vi "testAssertConnectorPanesMatchExpectedMissingFails.vi"(8 "error in (no error)":errorcluster, 11 "TestCase in":refnum<class "VeriStandTestUtilitiesTests.lvclass">) -> (0 "error out":errorcluster, 3 "TestCase out":refnum<class "VeriStandTestUtilitiesTests.lvclass">)   [LabVIEW 2027, in "VeriStandTestUtilitiesTests.lvclass"]
uses:
  VeriStandTestUtilitiesTests.lvclass
  <userlib>/_OpenG.lib/file/file.llb/Build Path - File Names Array - path__ogtk.vi
  <vilib>/addons/_JKI Toolkits/VI Tester/TestCase.llb/TestCase.lvclass
  Source/VeriStandTestUtilities/VeriStandTestUtilities.lvlib
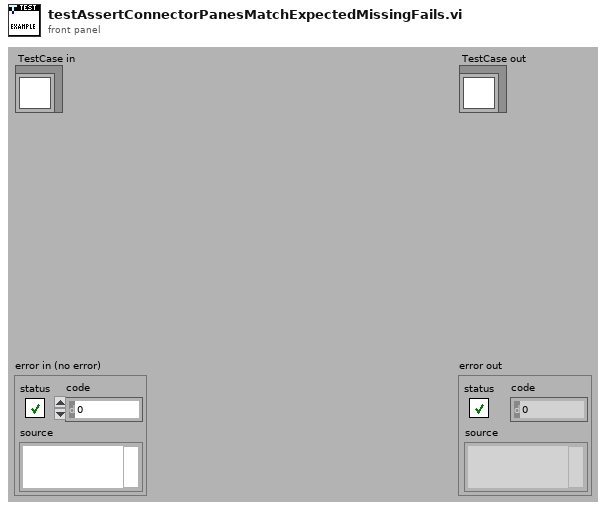
[diagram p1: front panel]
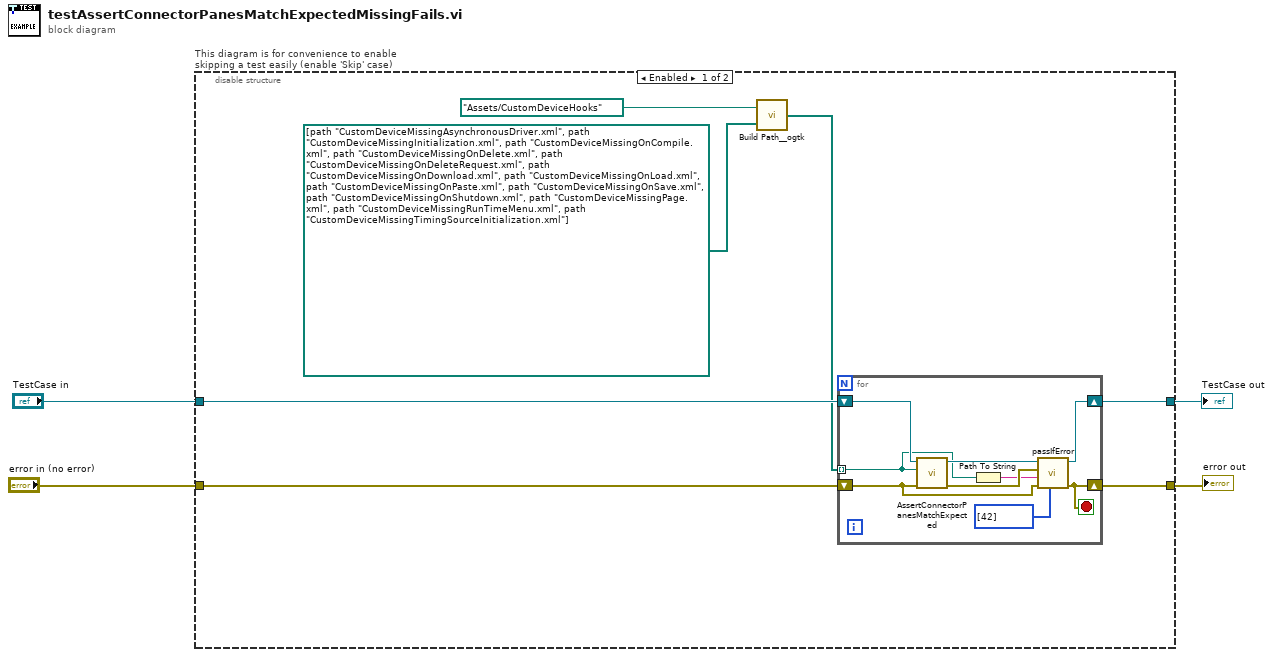
[diagram p0: block diagram]
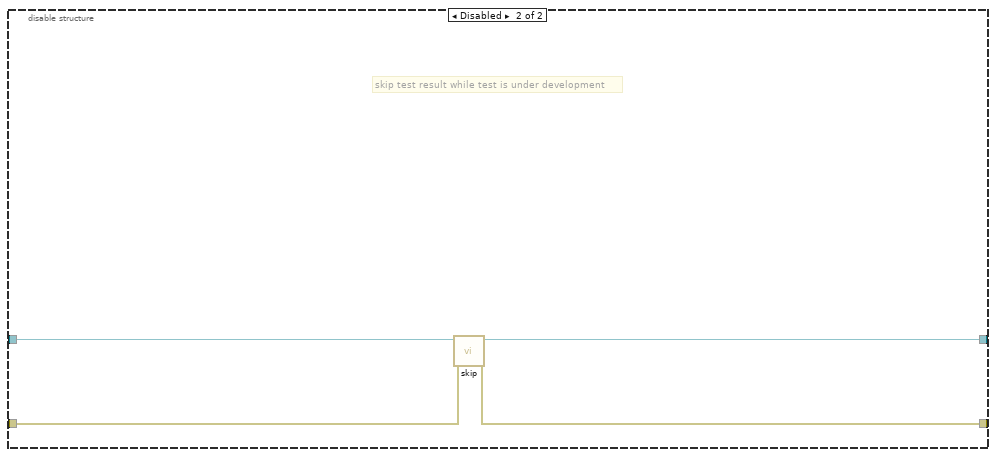
[diagram p2: hidden frame]
diagram:
  n1 = disable-structure "This diagram is for convenience to enable skipping a test easily (enable 'Skip' case)" shown="Enabled" {
    disable-tunnel: "TestCase in" -> [w9 w24]
    disable-tunnel: [w8 w22] -> w1
    disable-tunnel: [w10 w23] -> w3
    disable-tunnel: "error in (no error)" -> [w11 w21]
    frame Enabled {
      n2 = call-poly <userlib>:"Build Path__ogtk.vi"("name or relative path"=path[] [path "CustomDeviceMissingAsynchronousDriver.xml", path "CustomDeviceMissingInitialization.xml", path "CustomDeviceMissingOnCompile.xml", path "CustomDeviceMissingOnDelete.xml", path "CustomDeviceMissingOnDeleteRequest.xml", path "CustomDeviceMissingOnDownload.xml", path "CustomDeviceMissingOnLoad.xml", path "CustomDeviceMissingOnPaste.xml", path "CustomDeviceMissingOnSave.xml", path "CustomDeviceMissingOnShutdown.xml", path "CustomDeviceMissingPage.xml", path "CustomDeviceMissingRunTimeMenu.xml", path "CustomDeviceMissingTimingSourceInitialization.xml"], "base path"=path "Assets/CustomDeviceHooks") -> ("appended path"=w6:path[])
      n3 = for {
        tunnel: w6 -> [w15] mode=indexing
        shift-right: [w12] -> w10
        shift-left: w11 -> [w18]
        shift-right: [w16] -> w8
        shift-left: w9 -> [w17]
        stop <- w12 stop-if-true
        n4 = call "AssertConnectorPanesMatchExpected.vi"("error in (no error)"=w18, "custom device xml path"=w15, "TestCase in"=w17) -> ("error out"=w19:errorcluster, "TestCase out"=w20:refnum<class "VeriStandTestUtilitiesTests.lvclass">)  [unwired: 7 in]
        n5 = Path To String(path=w15) -> (string=w14:string)
        n6 = call-dynamic "passIfError.vi"("passing error codes (default = any error code)"=i32[] [42], "error in (no error)"=w18, "task (\"\")"=w14, "error"=w19, "TestCase in"=w20) -> ("error out"=w12:errorcluster, "TestCase out"=w16:refnum<class "VeriStandTestUtilitiesTests.lvclass">)  [unwired: 5 in]
      }
    }
    frame Disabled {
      # "skip test result while test is under development"
      n7 = call <vilib>:"skip.vi"("error in (no error)"=w21, "TestCase in"=w24) -> ("error out"=w23:errorcluster, "TestCase out"=w22:refnum<class "VeriStandTestUtilitiesTests.lvclass">)  [unwired: 8 in]
    }
  }
  "error out" <- w3
  "TestCase out" <- w1
